vi "Display Console View.vi"(8 "error in (no error)":errorcluster, 11 "View Model":T2) -> (0 "error out":errorcluster)   [LabVIEW 2017]
doc: "GUI process for operate Display Console"
uses:
  View Model/Controls/View Model.ctl
  Configuration/Controls/Config Model.ctl
  Configuration/Controls/Config Data.ctl
  Error Handler/Controls/Error Model.ctl
  Error Handler/Controls/Error Data.ctl
  Error Handler/Controls/Error Type.ctl
  View Model/Controls/Shared Model.ctl
  Elevator Controller/Controls/Elevator Model.ctl
  Elevator Controller/Controls/Elevator Location.ctl
  Elevator Controller/Controls/Elevator CMD Data.ctl
  Elevator Controller/Controls/Elevator Commands.ctl
  Elevator Controller/Controls/Elevator Overhead.ctl
  Elevator Controller/Controls/Elevator States.ctl
panel:
  out "Emergency":bool
  out "Door Open":bool
  out "Down":bool
  out "Up":bool
  out "Elevator Location":T1
  out "Timing":dbl
  # "[Covers: UI3C]"
  # "[Covers: UI3A]"
  # "[Covers: UI3D]"
  # "Elevator Direction"
  # "[Covers: UI2A1]"
  # "[Covers: UI3B]"
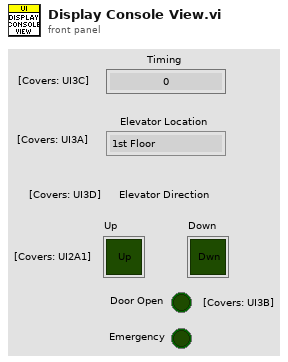
[diagram p1: front panel]
types:
  T1 = typedef "Elevator Location.ctl" = enum16{"1st Floor", "2nd Floor", "3rd Floor", "4th Floor"}
  T2 = typedef "View Model.ctl" = cluster{"Config Model":T3, "Error Model":T4, "Shared Model":T5, "Elevator Model":T6}
  T3 = typedef "Config Model.ctl" = cluster{"Config Change":refnum<user-event>, "Config Data":refnum<data-value>}
  T4 = typedef "Error Model.ctl" = cluster{"Error Event":refnum<user-event>}
  T5 = typedef "Shared Model.ctl" = cluster{"Stop Event":refnum<user-event>, "Stop DVR":refnum<data-value>}
  T6 = typedef "Elevator Model.ctl" = cluster{"Motion Change":refnum<user-event>, "Direction Change":refnum<user-event>, "Door Position Change":refnum<user-event>, "Emergency Change":refnum<user-event>, "Floor Change":refnum<user-event>, "Elevator CMD":refnum<user-event>, "Controller Overhead":refnum<data-value>}
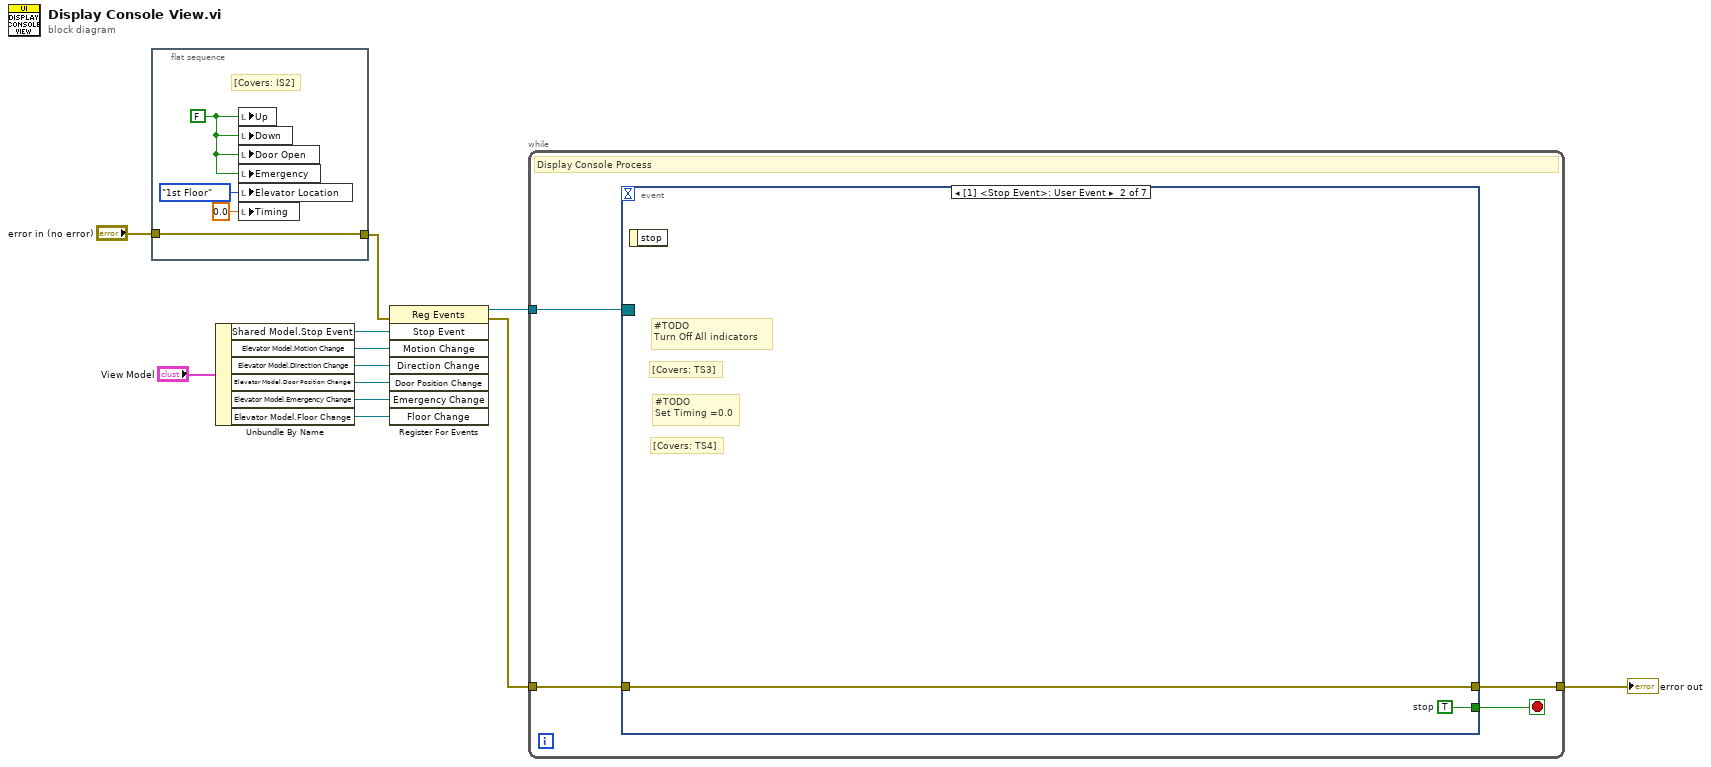
[diagram p0: block diagram]
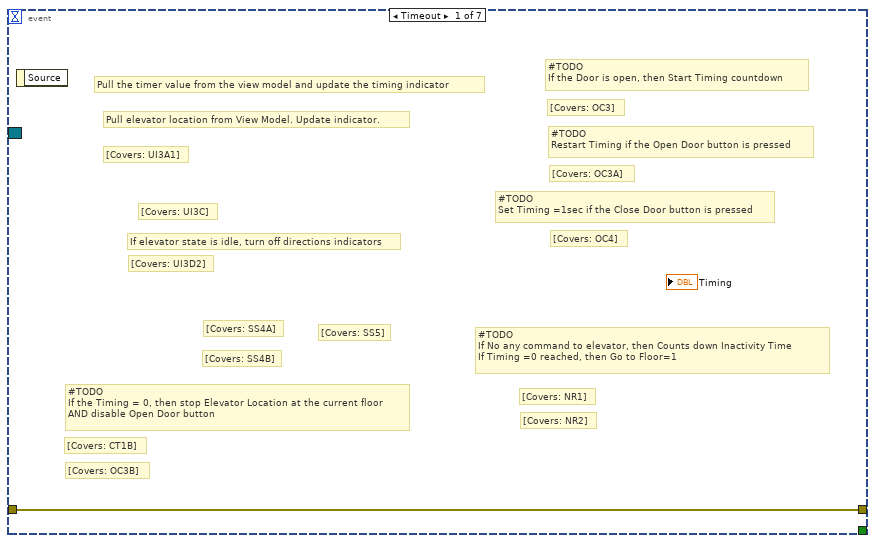
[diagram p2: hidden frame]
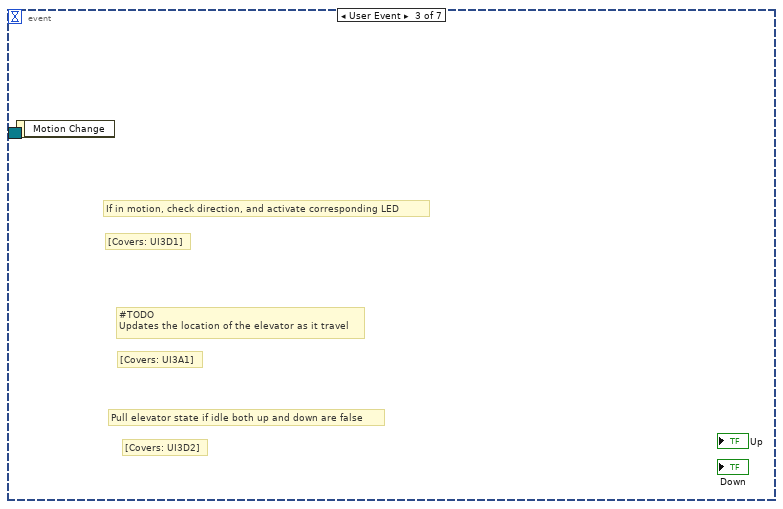
[diagram p3: hidden frame]
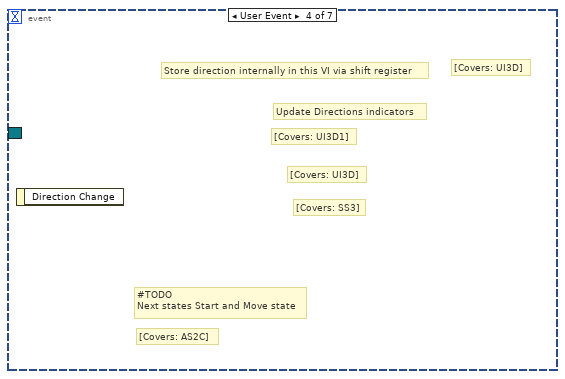
[diagram p4: hidden frame]
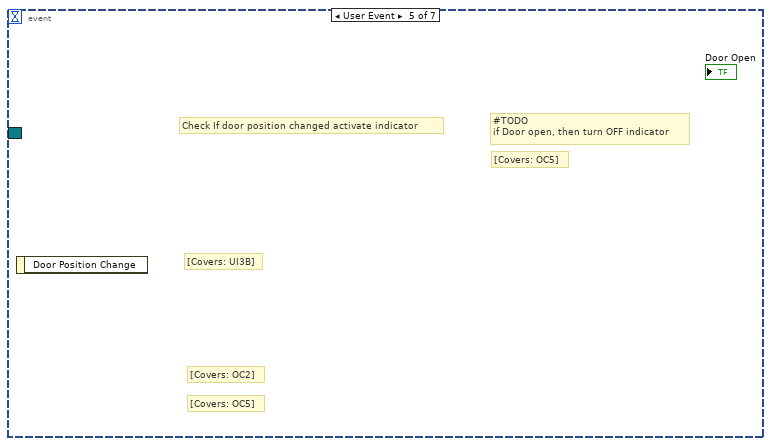
[diagram p5: hidden frame]
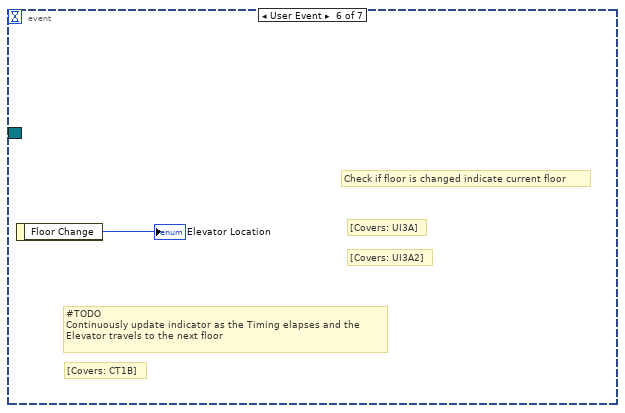
[diagram p6: hidden frame]
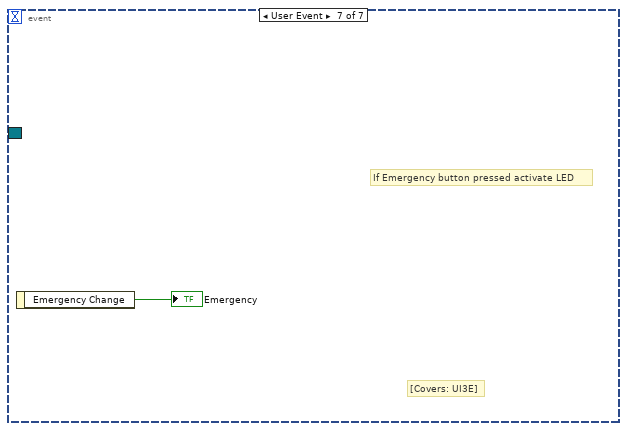
[diagram p7: hidden frame]
diagram:
  n1 = flat-sequence {
    tunnel: "error in (no error)" -> [w16]
    tunnel: [w16] -> w2
    frame #0 {
      w13 = FALSE ("Up")
      # "[Covers: IS2]"
      n2 = local write "Up"(w13) -> ()
      n3 = local write "Down"(w13) -> ()
      n4 = local write "Door Open"(w13) -> ()
      n5 = local write "Emergency"(w13) -> ()
      n6 = local write "Elevator Location"(Elevator_Location."1st Floor" ("Elevator Location")) -> ()
      n7 = local write "Timing"(0.0 ("Timing")) -> ()
    }
  }
  n8 = Unbundle By Name("View Model") -> ("Shared Model.Stop Event"=w12:refnum<user-event>, "Elevator Model.Motion Change"=w11:refnum<user-event>, "Elevator Model.Direction Change"=w7:refnum<user-event>, "Elevator Model.Door Position Change"=w6:refnum<user-event>, "Elevator Model.Emergency Change"=w5:refnum<user-event>, "Elevator Model.Floor Change"=w4:refnum<user-event>)
  n9 = register-events(error in=w2, w12, w11, w7, w6, w5, w4) -> (reference out=w10:refnum<event-registration>, error out=w1:errorcluster)  [unwired: 1 in]
  n10 = while {
    tunnel: w10 -> [w20]
    tunnel: w1 -> [w19]
    tunnel: [w18] -> w8
    stop <- w17 stop-if-true
    # "Display Console Process"
    n11 = event shown="[1] <Stop Event>: User Event" {
      selector: w20 -> [_ _ _ _ _ _ _]
      dyn-events: _ -> [_ _ _ _ _ _ _]
      timeout: _ -> [_ _ _ _ _ _ _]
      tunnel: w19 -> [w21 w22 _ _ _ _ _]
      tunnel: [w21 w22 _ _ _ _ _] -> w18
      tunnel: [_ w23 _ _ _ _ _] -> w17
      event Timeout {
        # "[Covers: NR2]"
        # "[Covers: NR1]"
        # "#TODO\nIf No any command to elevator, then Counts down Inactivity Time\nIf Timing =0 reached, then Go to Floor=1"
        # "[Covers: OC4]"
        # "#TODO\nSet Timing =1sec if the Close Door button is pressed"
        # "[Covers: OC3B]"
        # "[Covers: OC3A]"
        # "#TODO\nRestart Timing if the Open Door button is pressed"
        # "[Covers: OC3]"
        # "#TODO\nIf the Door is open, then Start Timing countdown"
        # "[Covers: CT1B]"
        # "#TODO\nIf the Timing = 0, then stop Elevator Location at the current floor\nAND disable Open Door button"
        # "[Covers: SS4B]"
        # "[Covers: SS5]"
        # "[Covers: SS4A]"
        # "[Covers: UI3D2]"
        # "If elevator state is idle, turn off directions indicators"
        # "[Covers: UI3A1]"
        # "Pull elevator location from View Model. Update indicator."
        # "[Covers: UI3C]"
        # "Pull the timer value from the view model and update the timing indicator"
        n12 = event-data() -> ()  [unwired: 1 in, 1 out]
      }
      event User Event {
        w23 = TRUE  # stop
        # "[Covers: TS4]"
        # "#TODO\nSet Timing =0.0"
        # "[Covers: TS3]"
        # "#TODO\nTurn Off All indicators"
        n13 = event-data() -> ()  [unwired: 1 in, 1 out]
      }
      event User Event {
        # "[Covers: UI3A1]"
        # "#TODO\nUpdates the location of the elevator as it travel"
        # "[Covers: UI3D2]"
        # "Pull elevator state if idle both up and down are false"
        # "[Covers: UI3D1]"
        # "If in motion, check direction, and activate corresponding LED"
        n14 = event-data() -> ()  [unwired: 1 in, 1 out]
      }
      event User Event {
        # "[Covers: AS2C]"
        # "#TODO\nNext states Start and Move state"
        # "[Covers: SS3]"
        # "[Covers: UI3D]"
        # "[Covers: UI3D1]"
        # "Update Directions indicators"
        # "[Covers: UI3D]"
        # "Store direction internally in this VI via shift register"
        n15 = event-data() -> ()  [unwired: 1 in, 1 out]
      }
      event User Event {
        # "[Covers: OC5]"
        # "#TODO\nif Door open, then turn OFF indicator"
        # "[Covers: OC5]"
        # "[Covers: OC2]"
        # "[Covers: UI3B]"
        # "Check If door position changed activate indicator"
        n16 = event-data() -> ()  [unwired: 1 in, 1 out]
      }
      event User Event {
        # "[Covers: CT1B]"
        # "#TODO\nContinuously update indicator as the Timing elapses and the\nElevator travels to the next floor"
        # "[Covers: UI3A2]"
        # "[Covers: UI3A]"
        # "Check if floor is changed indicate current floor"
        n17 = event-data() -> ("Floor Change"=→"Elevator Location":T1)  [unwired: 1 in]
      }
      event User Event {
        # "[Covers: UI3E]"
        # "If Emergency button pressed activate LED"
        n18 = event-data() -> ("Emergency Change"=→"Emergency":bool)  [unwired: 1 in]
      }
    }
  }
  "error out" <- w8
